vi "6332B关闭.vi"(8 "错误输入":errorcluster, 11 "VISA资源名称":refnum<visa-resource-name>) -> (0 "error out":errorcluster)   [LabVIEW 2021]
uses:
  <instrlib>/IT6300/IT6300.lvlib
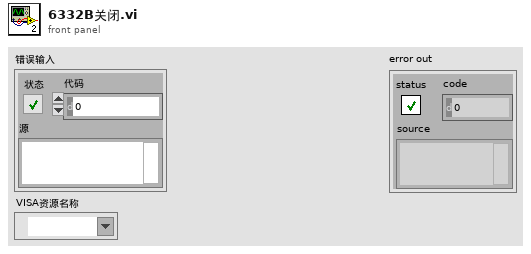
[diagram p1: front panel]
types:
  T1 = cluster{"Channel1":bool, "Channel2":bool, "Channel3":bool}
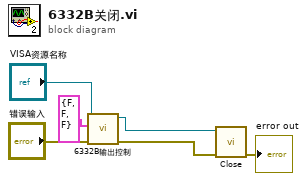
[diagram p0: block diagram]
diagram:
  n1 = call "6332B输出控制.vi"("错误输入"="错误输入", "Choose Channel"=T1 {"Channel1"=FALSE, "Channel2"=FALSE, "Channel3"=FALSE}, "VISA资源名称"="VISA资源名称") -> ("错误输出"=w4:errorcluster, "VISA资源名称输出"=w5:refnum<visa-resource-name>)  [unwired: 7 in]
  n2 = call <instrlib>:"Close.vi"("error in (no error)"=w4, "VISA resource name"=w5) -> ("error out"=→"error out":errorcluster)  [unwired: 9 in]
